vi "PS Control.vi"() -> ()   [LabVIEW 2020]
panel:
  out "Power Supply State":T1(ring)
  out "Output Cluster":T2 {"MaxLambdaCurrent [A]" format="%.2f"; "LambdaRates [A/min]" format="%.5e"; "MaxNormalCurrent [A]" format="%.2f"; "StabilitySetting [%]" format="%.2f"; "FieldCurrentRatio [T/A]" format="%.2f"; "SwitchWaitTime [s]" format="%.2f"; "SwitchHtrCurrent [mA]" format="%.2f"; "TrainRates [A/min]" format="%.5e"; "NormalRates [A/min]" format="%.5e"; "Breakpts [A]" format="%.5e"}
  in  "Local Enable":bool
  in  "Lambda Mode":bool
  in  "Training Mode":bool
  out "Lambda":bool
  out "Train":bool
  out "Persistent Field":dbl format="%.4f"
  out "Persistence Status":string
  out "Persistent":bool
  in  "Return from persistence":bool
  in  "Make Persistent":bool
  in  "Ramp to Zero":bool
  in  "Hold":bool
  in  "Ramp to Setpoint":bool
  in  "Slew Rate [T/min]":dbl min=0.0 max=5.0 step=0.1 format="%.5f"
  in  "Setpoint [T]":dbl format="%.5f"
  out "Magnet \nVoltage":dbl format="%.2f"
  out "Field [T]":dbl format="%.4f"
  out "Switch Heater Error":bool
  out "Switch heater \nconfirmed":bool
  out "Switch Heater":bool
  in  "VISA session":refnum<visa-resource-name>="GPIB0::25::INSTR"
  in  "stop":bool
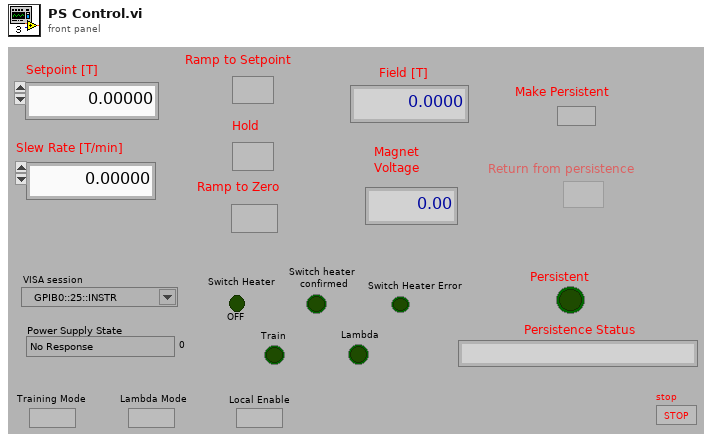
[diagram p1: front panel]
types:
  T1 = enum16{"No Response", "Ramping to programmed field ", "Holding at programmed field", "Paused", "Ramp Manual Up", "Ramp Manual Down", "Ramping to Zero", "QUENCH", "Heating Persistence Switch", "At Zero Current"}
  T2 = cluster{"Breakpts [A]":dbl[], "NormalRates [A/min]":dbl[], "TrainRates [A/min]":dbl[], "SwitchHtrCurrent [mA]":dbl, "SwitchWaitTime [s]":dbl, "FieldCurrentRatio [T/A]":dbl, "StabilitySetting [%]":dbl, "MaxNormalCurrent [A]":dbl, "Magnet ID":string, "LambdaRates [A/min]":dbl[], "MaxLambdaCurrent [A]":dbl}
  T3 = enum16{"Normal", "Train", "Lambda", "Train & Lambda"}
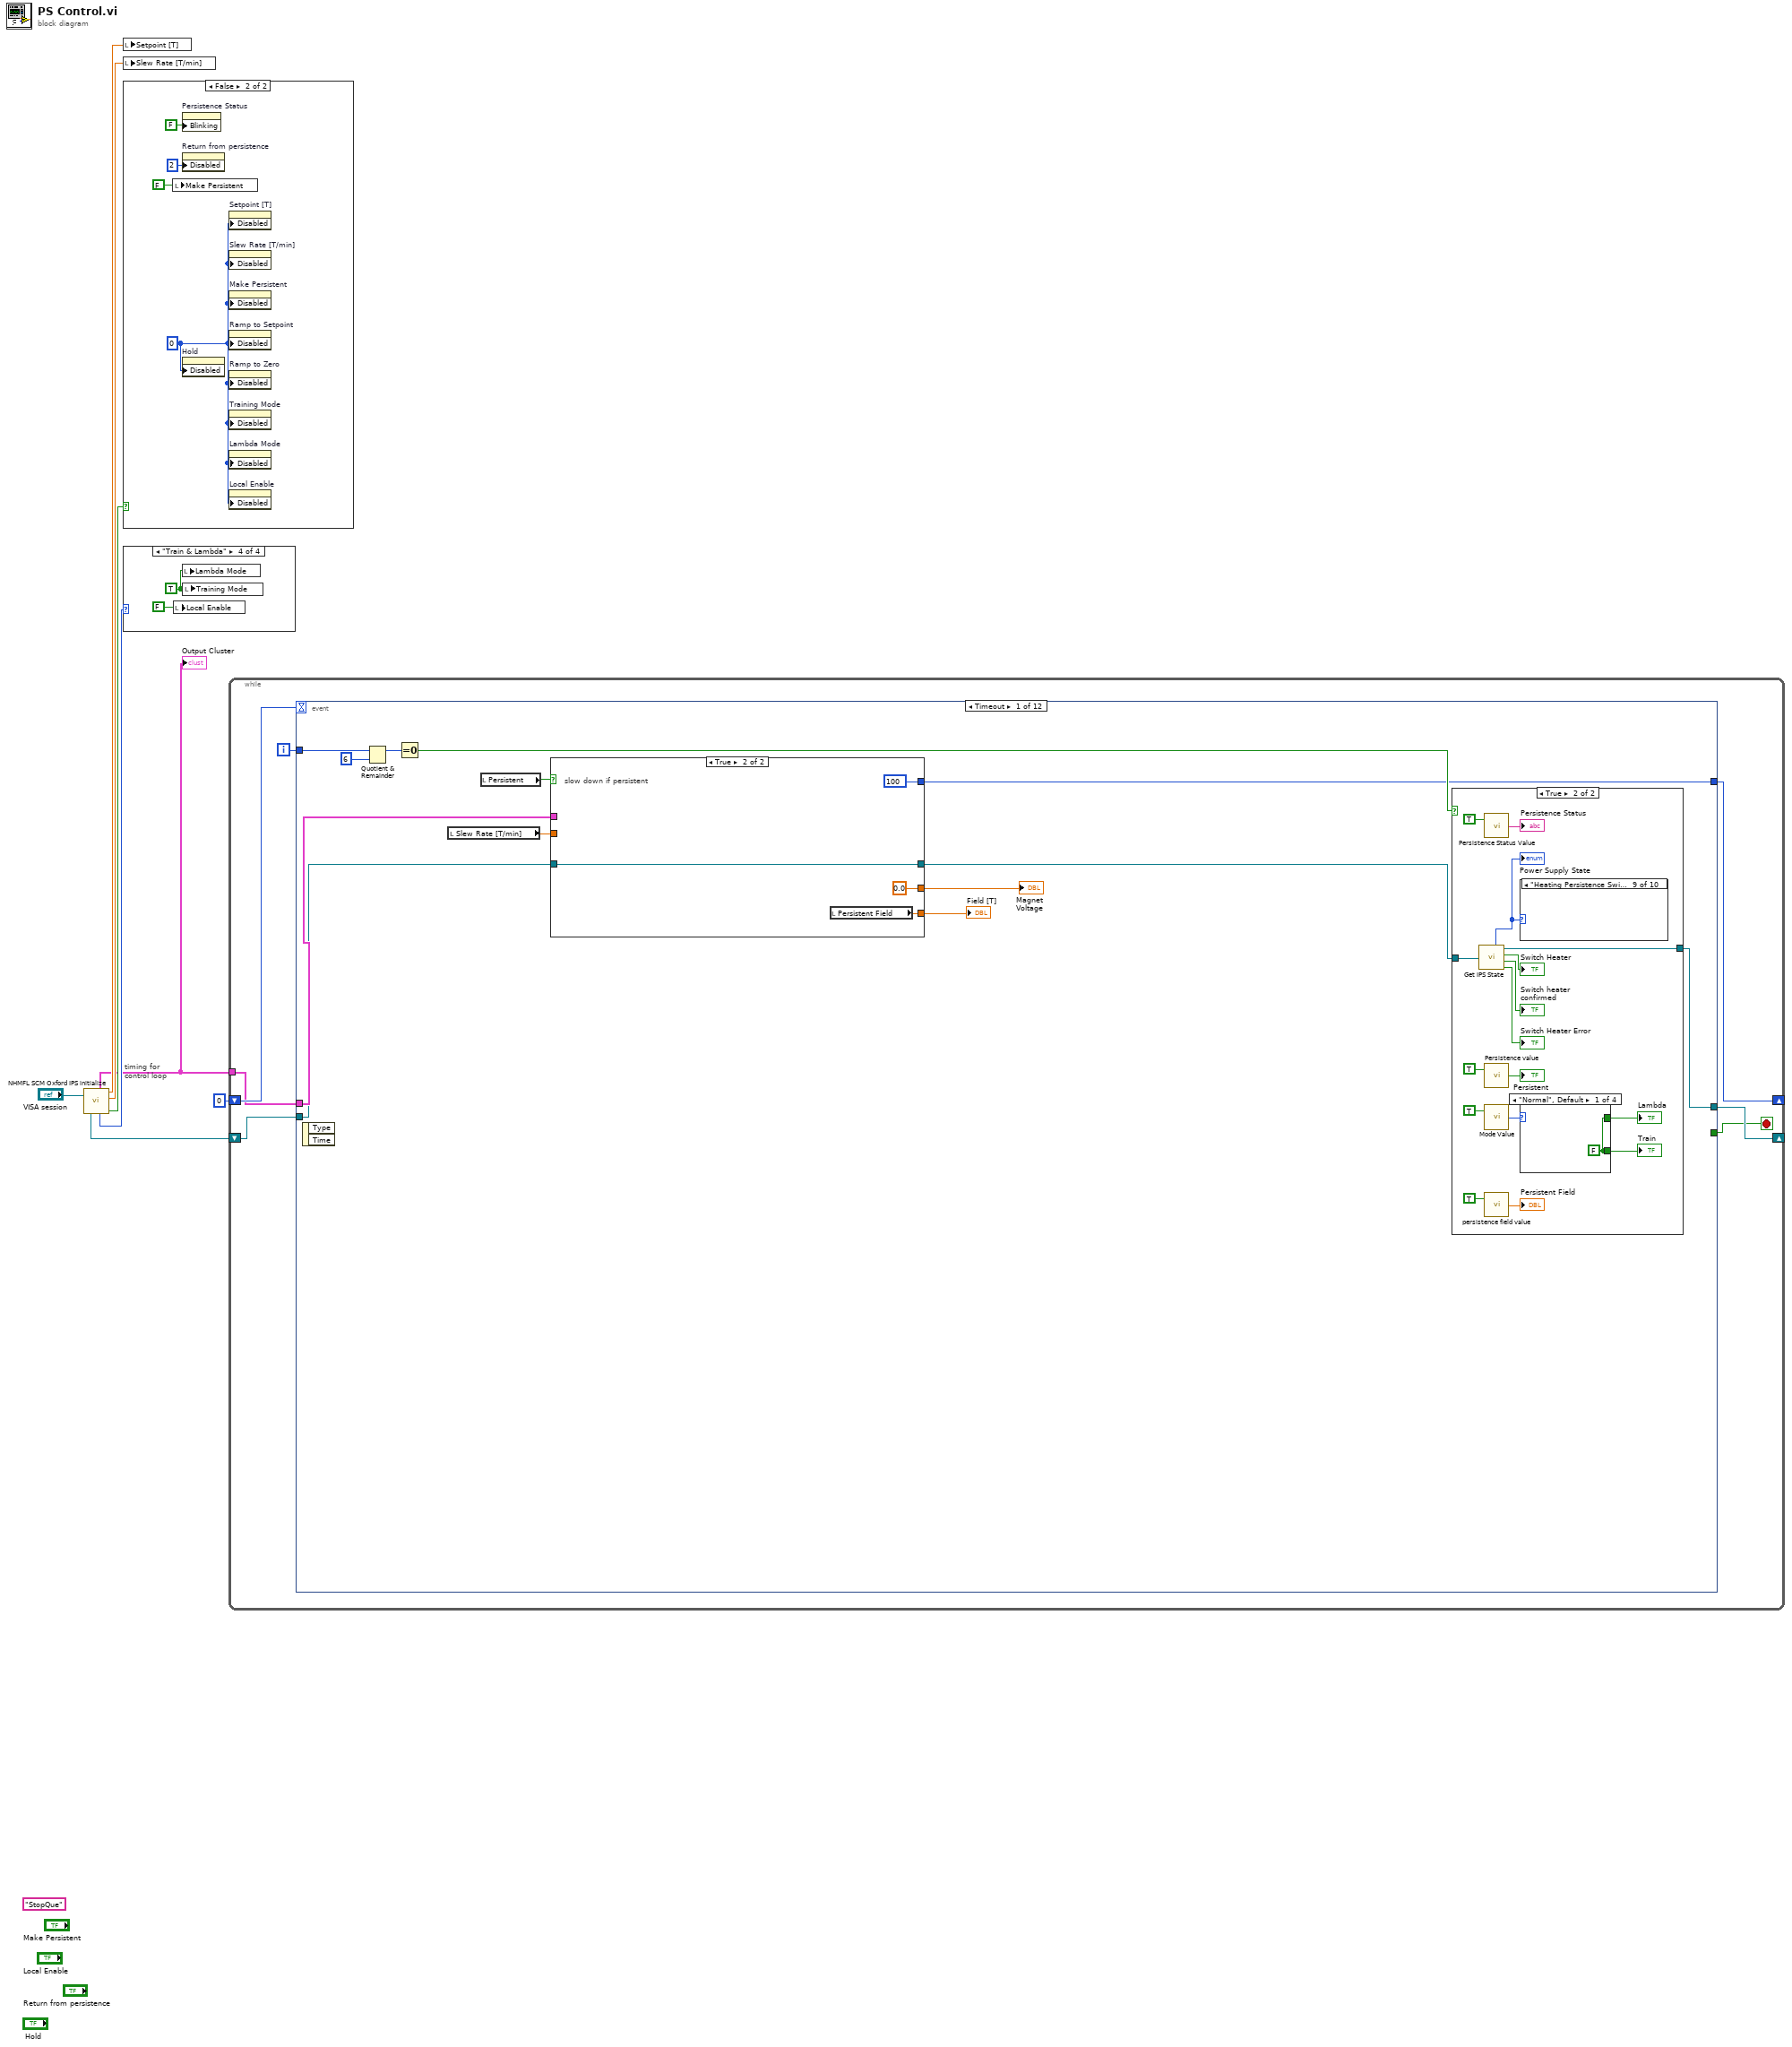
[diagram p0: block diagram]
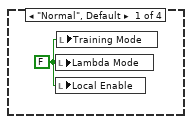
[diagram p2: hidden frame]
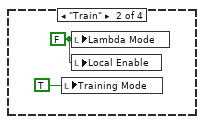
[diagram p3: hidden frame]
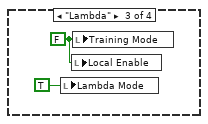
[diagram p4: hidden frame]
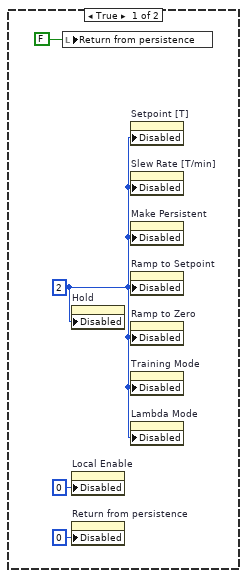
[diagram p5: hidden frame]
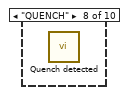
[diagram p14: hidden frame]
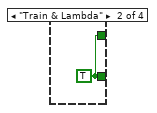
[diagram p16: hidden frame]
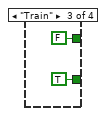
[diagram p17: hidden frame]
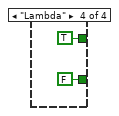
[diagram p18: hidden frame]
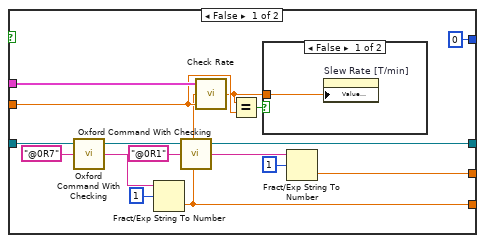
[diagram p19: hidden frame]
diagram:
  (unwired) "StopQue" ("name (unnamed)")
  # "timing for \ncontrol loop"
  n1 = call "NHMFL SCM Oxford IPS initialize.vi"("VISA session"="VISA session") -> ("dup VISA session"=w3:refnum<visa-resource-name>, "Output Cluster"=w2:T2, "Mode Out"=w5:T3, "Programmed Field"=w8:dbl, "Ramp Rate"=w4:dbl, "Persistent"=w6:bool)  [unwired: 1 out]
  "Output Cluster" <- w2
  n2 = local write "Setpoint [T]"(w8) -> ()
  n3 = local write "Slew Rate [T/min]"(w4) -> ()
  n4 = case shown="False" w6 {
    frame True {
      w10 = 2
      n5 = local write "Return from persistence"(FALSE ("Return from persistence")) -> ()
      n6 = property on="Hold" class="Bool (strict)"("Disabled"=w10) -> ()  [unwired: 2 in, 2 out]
      n7 = property on="Local Enable" class="Bool (strict)"("Disabled"=u8 0) -> ()  [unwired: 2 in, 2 out]
      n8 = property on="Return from persistence" class="Bool (strict)"("Disabled"=u8 0) -> ()  [unwired: 2 in, 2 out]
      n9 = property on="Setpoint [T]" class="DigNum (strict)"("Disabled"=w10) -> ()  [unwired: 2 in, 2 out]
      n10 = property on="Slew Rate [T/min]" class="DigNum (strict)"("Disabled"=w10) -> ()  [unwired: 2 in, 2 out]
      n11 = property on="Make Persistent" class="Bool (strict)"("Disabled"=w10) -> ()  [unwired: 2 in, 2 out]
      n12 = property on="Ramp to Setpoint" class="Bool (strict)"("Disabled"=w10) -> ()  [unwired: 2 in, 2 out]
      n13 = property on="Ramp to Zero" class="Bool (strict)"("Disabled"=w10) -> ()  [unwired: 2 in, 2 out]
      n14 = property on="Training Mode" class="Bool (strict)"("Disabled"=w10) -> ()  [unwired: 2 in, 2 out]
      n15 = property on="Lambda Mode" class="Bool (strict)"("Disabled"=w10) -> ()  [unwired: 2 in, 2 out]
    }
    frame False {
      w14 = 0
      n16 = local write "Make Persistent"(FALSE ("Return from persistence")) -> ()
      n17 = property on="Persistence Status" class="Str"("Blinking"=FALSE) -> ()  [unwired: 2 in, 2 out]
      n18 = property on="Return from persistence" class="Bool (strict)"("Disabled"=u8 2) -> ()  [unwired: 2 in, 2 out]
      n19 = property on="Hold" class="Bool (strict)"("Disabled"=w14) -> ()  [unwired: 2 in, 2 out]
      n20 = property on="Setpoint [T]" class="DigNum (strict)"("Disabled"=w14) -> ()  [unwired: 2 in, 2 out]
      n21 = property on="Slew Rate [T/min]" class="DigNum (strict)"("Disabled"=w14) -> ()  [unwired: 2 in, 2 out]
      n22 = property on="Make Persistent" class="Bool (strict)"("Disabled"=w14) -> ()  [unwired: 2 in, 2 out]
      n23 = property on="Ramp to Setpoint" class="Bool (strict)"("Disabled"=w14) -> ()  [unwired: 2 in, 2 out]
      n24 = property on="Ramp to Zero" class="Bool (strict)"("Disabled"=w14) -> ()  [unwired: 2 in, 2 out]
      n25 = property on="Training Mode" class="Bool (strict)"("Disabled"=w14) -> ()  [unwired: 2 in, 2 out]
      n26 = property on="Lambda Mode" class="Bool (strict)"("Disabled"=w14) -> ()  [unwired: 2 in, 2 out]
      n27 = property on="Local Enable" class="Bool (strict)"("Disabled"=w14) -> ()  [unwired: 2 in, 2 out]
    }
  }
  n28 = case shown="\"Train & Lambda\"" w5 {
    frame "Normal", Default {
      w17 = FALSE ("Training Mode")
      n29 = local write "Lambda Mode"(w17) -> ()
      n30 = local write "Local Enable"(w17) -> ()
      n31 = local write "Training Mode"(w17) -> ()
    }
    frame "Train" {
      w19 = FALSE
      n32 = local write "Training Mode"(TRUE) -> ()
      n33 = local write "Lambda Mode"(w19) -> ()
      n34 = local write "Local Enable"(w19) -> ()
    }
    frame "Lambda" {
      w20 = FALSE
      n35 = local write "Lambda Mode"(TRUE) -> ()
      n36 = local write "Local Enable"(w20) -> ()
      n37 = local write "Training Mode"(w20) -> ()
    }
    frame "Train & Lambda" {
      w22 = TRUE
      n38 = local write "Local Enable"(FALSE) -> ()
      n39 = local write "Lambda Mode"(w22) -> ()
      n40 = local write "Training Mode"(w22) -> ()
    }
  }
  n41 = while {
    tunnel: w2 -> [w28]
    shift-right: [w27] -> _
    shift-left: w3 -> [w30]
    shift-right: [w25] -> _
    shift-left: 0 ("y") -> [w29]
    i -> [w26]
    stop <- w24 stop-if-true
    n42 = event shown="[0] Timeout" {
      selector: _ -> [_ _ _ _ _ _ _ _ _ _ _ _]
      dyn-events: _ -> [_ _ _ _ _ _ _ _ _ _ _ _]
      timeout: w29 -> [_ w88 w91 w144 w170 w193 w243 w256 w272 w281 w287 w293]
      tunnel: w30 -> [w38 w89 w93 w145 w174 w196 w248 w261 w275 w284 w290 w295]
      tunnel: [_ w90 _ _ _ _ _ _ _ _ _ _] -> w24
      tunnel: w28 -> [w39 _ _ _ w173 w198 w246 w259 w279 _ _ _]
      tunnel: [w36 w89 w92 w145 w171 w194 w244 w257 w273 w282 w288 w294] -> w27
      tunnel: w26 -> [w35 _ _ _ _ _ _ _ _ _ _ _]
      tunnel: [w32 w88 w91 w144 w170 w193 w243 w256 w272 w281 w287 w293] -> w25
      event Timeout {
        n43 = event-data() -> ()  [unwired: 1 in, 2 out]
        n44 = Quotient & Remainder(x=w35, y=6) -> (x-y*floor(x/y)=w31:i32)  [unwired: 1 out]
        n45 = Equal To 0?(x=w31) -> (x = 0?=w33:bool)
        n46 = local read "Slew Rate [T/min]"() -> (w41:dbl)
        n47 = local read "Persistent"() -> (w40:bool)
        n48 = case shown="True" w40 {
          tunnel: w38 -> [w69 w85]
          tunnel: [w79 w87] -> w43
          tunnel: [w80 0.0] -> w42
          tunnel: w39 -> [w82 _]
          tunnel: w41 -> [w81 _]
          tunnel: [w68 w85] -> w37
          tunnel: [0 ("y") 100 ("y")] -> w32
          frame False {
            n49 = call "Oxford Command With Checking.vi"("Command"="@0R7", "VISA session"=w69) -> ("String Read"=w75:string, "dup VISA session"=w70:refnum<visa-resource-name>)  [unwired: 1 in, 1 out]
            n50 = Fract/Exp String To Number(string=w75, offset=1) -> (number=w79:dbl)  [unwired: 2 in, 1 out]
            n51 = call "Oxford Command With Checking.vi"("Command"="@0R1", "VISA session"=w70) -> ("String Read"=w72:string, "dup VISA session"=w68:refnum<visa-resource-name>)  [unwired: 1 in, 1 out]
            n52 = call "Check Rate.vi"("Rate"=w81, "Field"=w79, "input cluster"=w82) -> ("Checked Rate"=w77:dbl)
            n53 = Equal?(x=w77, y=w81) -> (x = y?=w78:bool)
            n54 = case shown="False" w78 {
              tunnel: w77 -> [w83 _]
              frame False {
                n55 = property on="Slew Rate [T/min]" class="DigNum (strict)"("Value (Signaling)"=w83) -> ()  [unwired: 2 in, 2 out]
              }
              frame True {
              }
            }
            n56 = Fract/Exp String To Number(string=w72, offset=1) -> (number=w80:dbl)  [unwired: 2 in, 1 out]
          }
          frame True {
            # "slow down if persistent"
            n57 = local read "Persistent Field"() -> (w87:dbl)
          }
        }
        "Field [T]" <- w43
        "Magnet \nVoltage" <- w42
        n58 = case shown="True" w33 {
          tunnel: w37 -> [w44 w46]
          tunnel: [w44 w45] -> w36
          frame False {
          }
          frame True {
            n59 = call "Get IPS State.vi"("VISA session"=w46) -> ("State"=w56:T1, "dup VISA session"=w45:refnum<visa-resource-name>, "Switch Heater"=→"Switch Heater":bool, "Switch heater \nconfirmed"=→"Switch heater \nconfirmed":bool, "Switch Heater Error"=→"Switch Heater Error":bool)  [unwired: 1 in]
            "Power Supply State" <- w56
            n60 = call "Persistence Status Value.vi"("Read/Write this vi"=TRUE) -> ("Persistence Status Out"=→"Persistence Status":string)  [unwired: 1 in]
            n61 = call "Persistence value.vi"("Read/Write this vi"=TRUE) -> ("Persistence Out"=→"Persistent":bool)  [unwired: 1 in]
            n62 = call "Mode Value.vi"("Read/Write this vi"=TRUE) -> ("Mode Out"=w53:T3)  [unwired: 1 in]
            n63 = call "persistence field value.vi"("Read/Write this vi"=TRUE) -> ("Persistent Field Out"=→"Persistent Field":dbl)  [unwired: 1 in]
            n64 = case shown="\"Heating Persistence Switch\"" w56 {
              frame "No Response", Default {
              }
              frame "Ramping to programmed field " {
              }
              frame "Holding at programmed field" {
              }
              frame "Paused" {
              }
              frame "Ramp Manual Up" {
              }
              frame "Ramp Manual Down" {
              }
              frame "Ramping to Zero" {
              }
              frame "QUENCH" {
                n65 = call "Quench detected.vi"() -> ()  [unwired: 1 out]
              }
              frame "Heating Persistence Switch" {
              }
              frame "At Zero Current" {
              }
            }
            n66 = case shown="\"Normal\", Default" w53 {
              tunnel: [w61 w62 TRUE FALSE] -> w54
              tunnel: [w61 w62 FALSE TRUE] -> w55
              frame "Normal", Default {
                w61 = FALSE
              }
              frame "Train & Lambda" {
                w62 = TRUE
              }
              frame "Train" {
              }
              frame "Lambda" {
              }
            }
            "Train" <- w54
            "Lambda" <- w55
          }
        }
      }
      event "stop": Value Change {
        n67 = event-data() -> ()  [unwired: 1 in, 5 out]
        n68 = call "PS PassWord.vi"() -> ("Password Correct"=w90:bool)  [unwired: 2 in]
      }
      event "Training Mode": Value Change {
        n69 = event-data() -> ()  [unwired: 1 in, 5 out]
        n70 = call "Mode Value.vi"("Read/Write this vi"=TRUE) -> ("Mode Out"=w94:T3)  [unwired: 1 in]
        n71 = case shown="False" "Training Mode" {
          tunnel: w94 -> [w99 w115]
          tunnel: w93 -> [w98 w114]
          tunnel: [w97 w113] -> w92
          frame False {
            n72 = case shown="\"Train\", Default" w99 {
              tunnel: w98 -> [w101 w107]
              tunnel: [w100 w106] -> w97
              frame "Train", Default {
                n73 = flat-sequence {
                  tunnel: w101 -> [w104]
                  tunnel: [w103] -> w100
                  frame #0 {
                    (unwired) T3."Normal" ("Mode In")
                    n74 = call "Mode Value.vi"("Read/Write this vi"=FALSE) -> ()  [unwired: 1 in, 1 out]
                  }
                  frame #1 {
                    n75 = call "Oxford Command With Checking.vi"("Command"="@0M1", "VISA session"=w104) -> ("dup VISA session"=w103:refnum<visa-resource-name>)  [unwired: 1 in, 2 out]
                  }
                }
              }
              frame "Train & Lambda" {
                n76 = flat-sequence {
                  tunnel: w107 -> [w111]
                  tunnel: [w110] -> w106
                  frame #0 {
                    n77 = call "Mode Value.vi"("Mode In"=T3."Lambda", "Read/Write this vi"=FALSE) -> ()  [unwired: 1 out]
                  }
                  frame #1 {
                    n78 = call "Oxford Command With Checking.vi"("Command"="@0M1", "VISA session"=w111) -> ("dup VISA session"=w110:refnum<visa-resource-name>)  [unwired: 1 in, 2 out]
                  }
                }
              }
            }
          }
          frame True {
            n79 = call "PS PassWord.vi"() -> ("Password Correct"=w116:bool)  [unwired: 2 in]
            n80 = case shown="False" w116 {
              tunnel: w115 -> [_ w121]
              tunnel: w114 -> [w117 w120]
              tunnel: [w117 w119] -> w113
              frame False {
                n81 = local write "Training Mode"(FALSE ("Train")) -> ()
              }
              frame True {
                n82 = case shown="\"Normal\", Default" w121 {
                  tunnel: w120 -> [w123 w134]
                  tunnel: [w122 w137] -> w119
                  frame "Normal", Default {
                    n83 = call "Mode Value.vi"("Mode In"=T3."Train", "Read/Write this vi"=FALSE) -> ("Mode Out"=w124:T3)
                    n84 = flat-sequence {
                      tunnel: w124 -> [_]
                      tunnel: w123 -> [w132]
                      tunnel: [w130] -> w122
                      frame #0 {
                        n85 = local read "Slew Rate [T/min]"() -> (w129:dbl)
                        n86 = local read "Field [T]"() -> (w128:dbl)
                        n87 = call "Check Rate.vi"("Rate"=w129, "Field"=w128) -> ("Checked Rate"=w127:dbl)  [unwired: 1 in]
                        n88 = local write "Slew Rate [T/min]"(w127) -> ()
                      }
                      frame #1 {
                        n89 = call "Oxford Command With Checking.vi"("Command"="@0M5", "VISA session"=w132) -> ("dup VISA session"=w130:refnum<visa-resource-name>)  [unwired: 1 in, 2 out]
                      }
                    }
                  }
                  frame "Lambda" {
                    n90 = call "Mode Value.vi"("Mode In"=T3."Train & Lambda", "Read/Write this vi"=FALSE) -> ("Mode Out"=w135:T3)
                    n91 = flat-sequence {
                      tunnel: w135 -> [_]
                      tunnel: w134 -> [w140]
                      tunnel: [w140] -> w133
                      frame #0 {
                        n92 = local read "Slew Rate [T/min]"() -> (w143:dbl)
                        n93 = local read "Field [T]"() -> (w142:dbl)
                        n94 = call "Check Rate.vi"("Rate"=w143, "Field"=w142) -> ("Checked Rate"=w141:dbl)  [unwired: 1 in]
                        n95 = local write "Slew Rate [T/min]"(w141) -> ()
                      }
                    }
                    n96 = call "Oxford Command With Checking.vi"("Command"="@0M5", "VISA session"=w133) -> ("dup VISA session"=w137:refnum<visa-resource-name>)  [unwired: 1 in, 2 out]
                  }
                }
              }
            }
          }
        }
      }
      event "Lambda Mode": Value Change {
        n97 = event-data() -> ()  [unwired: 1 in, 5 out]
        n98 = call "Mode Value.vi"("Read/Write this vi"=TRUE) -> ("Mode Out"=w146:T3)  [unwired: 1 in]
        n99 = case shown="True" "Lambda Mode" {
          tunnel: w146 -> [w149 w154]
          frame False {
            n100 = case shown="\"Lambda\", Default" w149 {
              frame "Lambda", Default {
                n101 = call "Mode Value.vi"("Mode In"=T3."Normal", "Read/Write this vi"=FALSE) -> ()  [unwired: 1 out]
              }
              frame "Train & Lambda" {
                n102 = call "Mode Value.vi"("Mode In"=T3."Train", "Read/Write this vi"=FALSE) -> ()  [unwired: 1 out]
              }
            }
          }
          frame True {
            n103 = call "PS PassWord.vi"() -> ("Password Correct"=w155:bool)  [unwired: 2 in]
            n104 = case shown="True" w155 {
              tunnel: w154 -> [_ w157]
              frame False {
                n105 = local write "Lambda Mode"(FALSE) -> ()
              }
              frame True {
                n106 = case shown="\"Normal\", Default" w157 {
                  frame "Train" {
                    n107 = call "Mode Value.vi"("Mode In"=T3."Train & Lambda", "Read/Write this vi"=FALSE) -> ("Mode Out"=w158:T3)
                    n108 = stacked-sequence {
                      tunnel: w158 -> [_]
                      frame #0 {
                        n109 = local read "Slew Rate [T/min]"() -> (w163:dbl)
                        n110 = local read "Field [T]"() -> (w162:dbl)
                        n111 = call "Check Rate.vi"("Rate"=w163, "Field"=w162) -> ("Checked Rate"=w161:dbl)  [unwired: 1 in]
                        n112 = local write "Slew Rate [T/min]"(w161) -> ()
                      }
                    }
                  }
                  frame "Normal", Default {
                    n113 = call "Mode Value.vi"("Mode In"=T3."Lambda", "Read/Write this vi"=FALSE) -> ("Mode Out"=w164:T3)
                    n114 = stacked-sequence {
                      tunnel: w164 -> [_]
                      frame #0 {
                        n115 = local read "Slew Rate [T/min]"() -> (w169:dbl)
                        n116 = local read "Field [T]"() -> (w168:dbl)
                        n117 = call "Check Rate.vi"("Rate"=w169, "Field"=w168) -> ("Checked Rate"=w167:dbl)  [unwired: 1 in]
                        n118 = local write "Slew Rate [T/min]"(w167) -> ()
                      }
                    }
                  }
                }
              }
            }
          }
        }
      }
      event "Local Enable": Value Change {
        n119 = event-data() -> ("NewVal"=w172:bool)  [unwired: 1 in, 4 out]
        n120 = case shown="True" w172 {
          tunnel: w174 -> [w177 w184]
          tunnel: w173 -> [_ w183]
          tunnel: [w175 w181] -> w171
          frame False {
            n121 = call "Oxford Command With Checking.vi"("Command"="@0C1", "VISA session"=w177) -> ("dup VISA session"=w176:refnum<visa-resource-name>)  [unwired: 1 in, 2 out]
            n122 = stacked-sequence {
              tunnel: w176 -> [w179]
              tunnel: [w179] -> w175
              frame #0 {
                n123 = local write "Local Enable"(FALSE ("Local Enable")) -> ()
              }
            }
          }
          frame True {
            n124 = call "PS PassWord.vi"() -> ("Password Correct"=w182:bool)  [unwired: 2 in]
            n125 = case shown="False" w182 {
              tunnel: w184 -> [w185 w189]
              tunnel: w183 -> [_ _]
              tunnel: [w185 w187] -> w181
              frame False {
                n126 = local write "Local Enable"(FALSE) -> ()
              }
              frame True {
                n127 = call "Oxford Command With Checking.vi"("Command"="@0C2", "VISA session"=w189) -> ("dup VISA session"=w188:refnum<visa-resource-name>)  [unwired: 1 in, 2 out]
                n128 = stacked-sequence {
                  tunnel: w188 -> [w191]
                  tunnel: [w191] -> w187
                  frame #0 {
                    n129 = local write "Local Enable"(TRUE) -> ()
                  }
                }
              }
            }
          }
        }
      }
      event "Setpoint [T]": Value Change {
        n130 = event-data() -> ()  [unwired: 1 in, 5 out]
        n131 = call "Mode Value.vi"("Read/Write this vi"=TRUE) -> ("Mode Out"=w200:T3)  [unwired: 1 in]
        n132 = case shown="\"Lambda\"" w200 {
          tunnel: "Setpoint [T]" -> [w205 w214 w224 w234]
          tunnel: w198 -> [w212 w222 w232 w242]
          tunnel: [w204 w216 w226 w236] -> w197
          frame "Normal", Default {
            n133 = Unbundle By Name(w212) -> ("MaxNormalCurrent [A]"=w210:dbl, "FieldCurrentRatio [T/A]"=w209:dbl)
            n134 = Multiply(x=w210, y=w209) -> (x*y=w211:dbl)
            n135 = Absolute Value(x=w205) -> (abs(x)=w208:dbl)
            n136 = In Range and Coerce(upper limit=w211, x=w208, lower limit=0.0) -> (coerced(x)=w206:dbl)  [unwired: 1 out]
            n137 = Sign(1:w205) -> (0:w203:dbl)
            n138 = Multiply(x=w206, y=w203) -> (x*y=w204:dbl)
          }
          frame "Train" {
            n139 = Unbundle By Name(w222) -> ("MaxNormalCurrent [A]"=w220:dbl, "FieldCurrentRatio [T/A]"=w219:dbl)
            n140 = Multiply(x=w220, y=w219) -> (x*y=w221:dbl)
            n141 = Absolute Value(x=w214) -> (abs(x)=w218:dbl)
            n142 = In Range and Coerce(upper limit=w221, x=w218, lower limit=0.0) -> (coerced(x)=w215:dbl)  [unwired: 1 out]
            n143 = Sign(1:w214) -> (0:w213:dbl)
            n144 = Multiply(x=w215, y=w213) -> (x*y=w216:dbl)
          }
          frame "Lambda" {
            n145 = Unbundle By Name(w232) -> ("MaxLambdaCurrent [A]"=w230:dbl, "FieldCurrentRatio [T/A]"=w229:dbl)
            n146 = Multiply(x=w230, y=w229) -> (x*y=w231:dbl)
            n147 = Absolute Value(x=w224) -> (abs(x)=w228:dbl)
            n148 = In Range and Coerce(upper limit=w231, x=w228, lower limit=0.0) -> (coerced(x)=w225:dbl)  [unwired: 1 out]
            n149 = Sign(1:w224) -> (0:w223:dbl)
            n150 = Multiply(x=w225, y=w223) -> (x*y=w226:dbl)
          }
          frame "Train & Lambda" {
            n151 = Unbundle By Name(w242) -> ("MaxLambdaCurrent [A]"=w240:dbl, "FieldCurrentRatio [T/A]"=w239:dbl)
            n152 = Multiply(x=w240, y=w239) -> (x*y=w241:dbl)
            n153 = Absolute Value(x=w234) -> (abs(x)=w238:dbl)
            n154 = In Range and Coerce(upper limit=w241, x=w238, lower limit=0.0) -> (coerced(x)=w235:dbl)  [unwired: 1 out]
            n155 = Sign(1:w234) -> (0:w233:dbl)
            n156 = Multiply(x=w235, y=w233) -> (x*y=w236:dbl)
          }
        }
        n157 = local write "Setpoint [T]"(w197) -> ()
        n158 = Format Into String(format string="@0J%+7.5f" ("Command String"), w197) -> (resulting string=w195:string)  [unwired: 2 in, 1 out]
        n159 = call "Oxford Command With Checking.vi"("Command"=w195, "VISA session"=w196) -> ("dup VISA session"=w194:refnum<visa-resource-name>)  [unwired: 1 in, 2 out]
      }
      event "Make Persistent": Value Change {
        # "make persistent routine"
        n160 = event-data() -> ()  [unwired: 1 in, 5 out]
        n161 = flat-sequence {
          tunnel: w248 -> [w253]
          tunnel: [w253] -> w247
          frame #0 {
            w255 = u8 2 ("Disabled")
            # "Disable controls"
            n162 = property on="Make Persistent" class="Bool (strict)"("Disabled"=w255) -> ()  [unwired: 2 in, 2 out]
            n163 = property on="Return from persistence" class="Bool (strict)"("Disabled"=w255) -> ()  [unwired: 2 in, 2 out]
            n164 = property on="Training Mode" class="Bool (strict)"("Disabled"=w255) -> ()  [unwired: 2 in, 2 out]
            n165 = property on="Lambda Mode" class="Bool (strict)"("Disabled"=w255) -> ()  [unwired: 2 in, 2 out]
            n166 = property on="Local Enable" class="Bool (strict)"("Disabled"=w255) -> ()  [unwired: 2 in, 2 out]
            n167 = property on="Persistence Status" class="Str"("Blinking"=TRUE) -> ()  [unwired: 2 in, 2 out]
            n168 = property on="Setpoint [T]" class="DigNum (strict)"("Disabled"=w255) -> ()  [unwired: 2 in, 2 out]
            n169 = property on="Hold" class="Bool (strict)"("Disabled"=w255) -> ()  [unwired: 2 in, 2 out]
            n170 = property on="Slew Rate [T/min]" class="DigNum (strict)"("Disabled"=w255) -> ()  [unwired: 2 in, 2 out]
            n171 = property on="Ramp to Setpoint" class="Bool (strict)"("Disabled"=w255) -> ()  [unwired: 2 in, 2 out]
            n172 = property on="Ramp to Zero" class="Bool (strict)"("Disabled"=w255) -> ()  [unwired: 2 in, 2 out]
          }
        }
        n173 = call "NML SCM IPS make persistent.vi"("VISA session"=w247, "Input Cluster"=w246) -> ("dup VISA session"=w245:refnum<visa-resource-name>)  [unwired: 3 out]
        n174 = flat-sequence {
          tunnel: w245 -> [w249]
          tunnel: [w249] -> w244
          frame #0 {
            # "enable return from persistence control"
            n175 = local write "Return from persistence"(FALSE ("Return from persistence")) -> ()
            n176 = property on="Return from persistence" class="Bool (strict)"("Disabled"=u8 0) -> ()  [unwired: 2 in, 2 out]
            n177 = property on="Persistence Status" class="Str"("Blinking"=FALSE) -> ()  [unwired: 2 in, 2 out]
          }
        }
      }
      event "Return from persistence": Value Change {
        # "run return from persistence vi"
        n178 = event-data() -> ()  [unwired: 1 in, 5 out]
        n179 = flat-sequence {
          tunnel: [w269] -> w260
          tunnel: w261 -> [w269]
          frame #0 {
            w271 = u8 2 ("Disabled")
            # "disable both controls (others should already be disabled)"
            n180 = property on="Persistence Status" class="Str"("Blinking"=TRUE) -> ()  [unwired: 2 in, 2 out]
            n181 = property on="Return from persistence" class="Bool (strict)"("Disabled"=w271) -> ()  [unwired: 2 in, 2 out]
            n182 = property on="Make Persistent" class="Bool (strict)"("Disabled"=w271) -> ()  [unwired: 2 in, 2 out]
          }
        }
        n183 = call "NML SCM IPS unpersistence.vi"("Input Cluster"=w259, "VISA session"=w260) -> ("dup VISA session"=w258:refnum<visa-resource-name>)  [unwired: 1 in, 2 out]
        n184 = flat-sequence {
          tunnel: w258 -> [w262]
          tunnel: [w262] -> w257
          frame #0 {
            w265 = u8 0 ("f")
            w267 = TRUE
            w264 = u8 0 ("Disabled")
            # "enable all controls except return from persistence \nand change rate back to normal"
            n185 = local write "Make Persistent"(FALSE ("Return from persistence")) -> ()
            n186 = local write "Hold"(w267) -> ()
            n187 = property on="Slew Rate [T/min]" class="DigNum (strict)"("Disabled"=w265) -> ()  [unwired: 2 in, 2 out]
            n188 = property on="Setpoint [T]" class="DigNum (strict)"("Disabled"=w265) -> ()  [unwired: 2 in, 2 out]
            n189 = property on="Ramp to Zero" class="Bool (strict)"("Disabled"=w265) -> ()  [unwired: 2 in, 2 out]
            n190 = property on="Ramp to Setpoint" class="Bool (strict)"("Disabled"=w265) -> ()  [unwired: 2 in, 2 out]
            n191 = property on="Hold" class="Bool (strict)"("Disabled"=w265) -> ()  [unwired: 2 in, 2 out]
            n192 = property on="Local Enable" class="Bool (strict)"("Disabled"=w264) -> ()  [unwired: 2 in, 2 out]
            n193 = property on="Make Persistent" class="Bool (strict)"("Disabled"=w264) -> ()  [unwired: 2 in, 2 out]
            n194 = property on="Training Mode" class="Bool (strict)"("Disabled"=w264) -> ()  [unwired: 2 in, 2 out]
            n195 = property on="Lambda Mode" class="Bool (strict)"("Disabled"=w264) -> ()  [unwired: 2 in, 2 out]
            n196 = property on="Persistence Status" class="Str"("Blinking"=FALSE) -> ()  [unwired: 2 in, 2 out]
            n197 = Not(x=w267) -> (.not. x?=w266:bool)
            n198 = local write "Ramp to Setpoint"(w266) -> ()
            n199 = local write "Ramp to Zero"(w266) -> ()
          }
        }
      }
      event "Slew Rate [T/min]": Value Change {
        n200 = event-data() -> ()  [unwired: 1 in, 5 out]
        n201 = local read "Field [T]"() -> (w278:dbl)
        n202 = call "Check Rate.vi"("Rate"="Slew Rate [T/min]", "Field"=w278, "input cluster"=w279) -> ("Checked Rate"=w276:dbl)
        n203 = local write "Slew Rate [T/min]"(w276) -> ()
        n204 = Format Into String(format string="@0T%+7.3f" ("Command String"), w276) -> (resulting string=w274:string)  [unwired: 2 in, 1 out]
        n205 = call "Oxford Command With Checking.vi"("Command"=w274, "VISA session"=w275) -> ("dup VISA session"=w273:refnum<visa-resource-name>)  [unwired: 1 in, 2 out]
      }
      event "Ramp to Setpoint": Value Change {
        w285 = TRUE
        n206 = event-data() -> ()  [unwired: 1 in, 5 out]
        n207 = local write "Ramp to Setpoint"(w285) -> ()
        n208 = call "Oxford Command With Checking.vi"("Command"="@0A1" ("Command String"), "VISA session"=w284) -> ("dup VISA session"=w282:refnum<visa-resource-name>)  [unwired: 1 in, 2 out]
        n209 = Not(x=w285) -> (.not. x?=w286:bool)
        n210 = local write "Hold"(w286) -> ()
        n211 = local write "Ramp to Zero"(w286) -> ()
      }
      event "Hold": Value Change {
        w291 = TRUE
        n212 = event-data() -> ()  [unwired: 1 in, 5 out]
        n213 = local write "Hold"(w291) -> ()
        n214 = call "Oxford Command With Checking.vi"("Command"="@0A0" ("Command String"), "VISA session"=w290) -> ("dup VISA session"=w288:refnum<visa-resource-name>)  [unwired: 1 in, 2 out]
        n215 = Not(x=w291) -> (.not. x?=w292:bool)
        n216 = local write "Ramp to Setpoint"(w292) -> ()
        n217 = local write "Ramp to Zero"(w292) -> ()
      }
      event "Ramp to Zero": Value Change {
        w297 = TRUE
        n218 = event-data() -> ()  [unwired: 1 in, 5 out]
        n219 = local write "Ramp to Zero"(w297) -> ()
        n220 = call "Oxford Command With Checking.vi"("Command"="@0A2" ("Command String"), "VISA session"=w295) -> ("dup VISA session"=w294:refnum<visa-resource-name>)  [unwired: 1 in, 2 out]
        n221 = Not(x=w297) -> (.not. x?=w298:bool)
        n222 = local write "Hold"(w298) -> ()
        n223 = local write "Ramp to Setpoint"(w298) -> ()
      }
    }
  }
